vi "AlliGator Load I-m-phi Dataset.vi"(5 "Image Type":string="Image", 7 "Bkgd Image Subtraction?":bool, 8 "error in (no error)":errorcluster, 9 "Control References":T1, 10 "Folder Path":path, 11 "AlliGator IV DVR in":refnum<data-value>) -> (0 "error out":errorcluster, 2 "Folder Path (dup)":path, 3 "AlliGator IV DVR out":refnum<data-value>, 4 "Result String":string)   [LabVIEW 2021, in "AlliGator Files.lvlib"]
doc: "Loads a FLI dataset comprised of an intensity and phase image (FLIMBox)."
uses:
  AlliGator Files.lvlib
  AlliGator Internal Variables v2.ctl
  <vilib>/vision/Image Controls.llb/IMAQ Image.ctl
  AlliGator Gate Image Set.ctl
  AlliGator FLI Dataset Type.ctl
  AlliGator Data Series Type.ctl
  AlliGator Dataset Channel.ctl
  AlliGator Gate Arithmetic.ctl
  AlliGator Displayed Image.ctl
  Image/Named ROI Description.ctl
  AlliGator Decay Metadata v3.ctl
  AlliGator Decay Background Subtraction Info.ctl
  AlliGator Baseline Subtraction Method.ctl
  Graphs/XY Graph/XY Graph Plot Shift Parameters.ctl
  Graphs/XY Graph/XY Graph Plot Shift Method.ctl
  AlliGator Decay Extrapolation Parameters.ctl
  Phasor/Calibration Phasor (m, phi).ctl
  Phasor/Phasor Reference Series.ctl
  Phasor/Phasor Calibration Map v2.ctl
  Phasor/Phasor (g, s).ctl
  AlliGator Raw Phasor Plot Data v4.ctl
  Phasor/Phasor Standard Deviation Options.ctl
  AlliGator Phasor Multi-Harmonic Data.ctl
  Phasor/Phasor Harmonic Data.ctl
  AlliGator Decay Fit Options & Parameters v2.ctl
  Fits/IRF(X)PSED/Decay Fit Options v2.ctl
  Fits/Decay Convolution/Decay Model.ctl
  Fits/Residual Type.ctl
  Fits/IRF(X)PSED/Fit Weights Type.ctl
  Fits/Non-linear Fitting Method v2.ctl
  Fits/Fit Calculation Method.ctl
  Fits/Non-linear Fitting Algorithm.ctl
  AlliGator Decay Fit Parameter Constraints 2.ctl
  Fits/IRF(X)PSED/Decay Fit Parameters In List.ctl
  Fits/IRF(X)PSED/MLE Baseline Offset Type.ctl
  AlliGator Decay Preprocessing Parameters.ctl
  Fits/IRF(X)PSED/Decay Fit Parameters & Derived Quantities List.ctl
  AlliGator Dataset Ctrl Refnums.ctl
  AlliGator After Loading Dataset Information.ctl
  AlliGator Gate Images Structure.ctl
  AlliGator I-m-phi Component List.ctl
  089290e1-c93f-4b42-a3f3-b2d44885c075.vi
  Arrays/n x n Kernel Convolution (SGL).vi
  Arrays/n x n Smoothen Array (SGL) v3.vi
  Arrays/n x n Kernel Convolution (SGL).vi/d0ebc029-cbaa-4c82-a58c-923c59c440da.vi
  Arrays/n x n Kernel Convolution (SGL).vi/b80d5e79-a0c8-46e2-aba9-3d60e0093a16.vi
  <vilib>/Analysis/2dsp.llb/Convolution.vi
  <vilib>/Analysis/2dsp.llb/2D Convolution (DBL).vi
  Arrays/Truncate Kernel.vi
  Arrays/Replace NaN by 0 (2D SGL).vi
  Arrays/n x n Smoothen Array (SGL) v3.vi/d0ebc029-cbaa-4c82-a58c-923c59c440da.vi
  Arrays/n x n Smoothen Array (SGL) v3.vi/b80d5e79-a0c8-46e2-aba9-3d60e0093a16.vi
  Arrays/Replace NaN by 0 (2D SGL).vi/df975b44-f6c5-4554-af30-980613d33749.vi
  Time/High Resolution Timing.vi
  Arrays/Compute n x n Kernel (SGL).vi
  <vilib>/Utility/error.llb/Simple Error Handler.vi
  <vilib>/Utility/error.llb/Error Cluster From Error Code.vi
  <vilib>/ErrorRing/Error Ring.xnode
  Image/Image.lvlib
  AlliGator Source Image.lvlib
  AlliGator GUI.lvlib
  GUI/GUI.lvlib
  Boolean/Boolean.lvlib
  Error/Error.lvlib
  Arrays/Arrays.lvlib
  Strings/Strings.lvlib
  Phasor/Phasor.lvlib
  AlliGator Decay Preprocessing.lvlib
  Graphs/XY Graph/XY Graph Add-Ons.lvlib
  AlliGator Phasor Graph.lvlib
  AlliGator Internal Variables.lvlib
  AlliGator Phasor Plot.lvlib
  Fits/Fits.lvlib
  AlliGator Decay Fit.lvlib
  AlliGator Decay Fit Parameter Map.lvlib
  AlliGator Settings.lvlib
  AlliGator Dual-Channel Datasets.lvlib
panel:
  out "# disposed images":i32
  out "# created images":i32
  # "see the AlliGator License on the block diagram (Ctrl+E or Window:Show Block Diagram)"
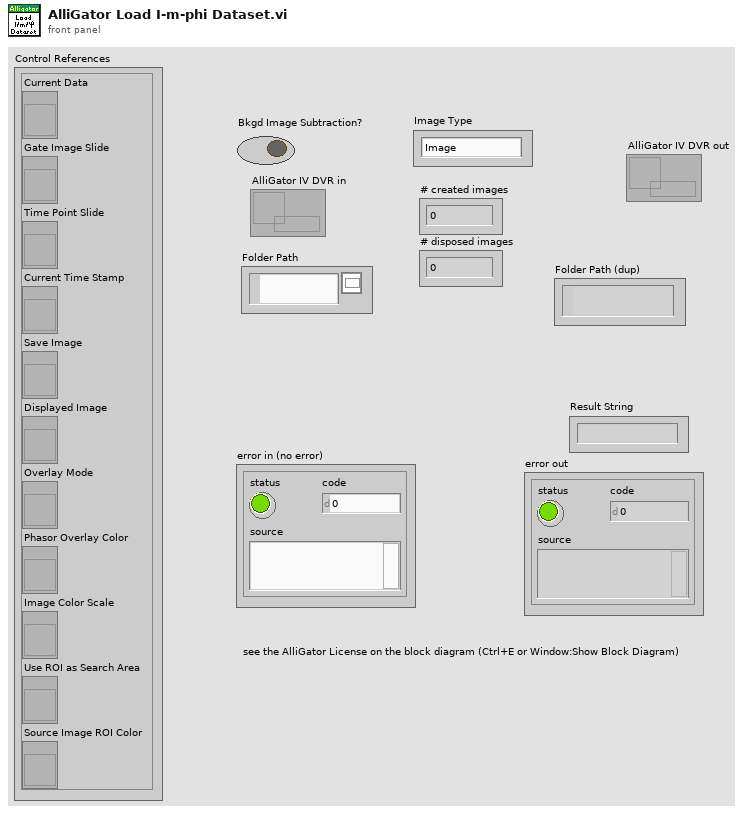
[diagram p1: front panel]
types:
  T1 = typedef "AlliGator GUI.lvlib/AlliGator Dataset Ctrl Refnums.ctl" = cluster{"Current Data":refnum<vi>, "Gate Image Slide":refnum<vi>, "Time Point Slide":refnum<vi>, "Current Time Stamp":refnum<vi>, "Save Image":refnum<vi>, "Displayed Image":refnum<vi>, "Overlay Mode":refnum<vi>, "Phasor Overlay Color":refnum<vi>, "Image Color Scale":refnum<vi>, "Use ROI as Search Area":refnum<vi>, "Source Image ROI Color":refnum<vi>}
  T2 = typedef "AlliGator Files.lvlib/AlliGator After Loading Dataset Information.ctl" = cluster{"Nanotime Gate Separation":dbl[unit], "Gate Width":dbl[unit], "Laser Period":dbl[unit], "Data Description":string, "# Pixel X":i32, "# Pixel Y":i32, "Gates to Use":cluster{"Start":u32, "End":u32}, "Gate Step":i32, "SYNC Period":dbl[unit], "X Binning":i32, "Y Binning":i32, "Gates to":bool, "Metadata":string, "Gate Image Exposure":dbl[unit], "Gate Image Integration":dbl[unit], "Macrotime Gate Separation":dbl[unit]}
  T3 = typedef "AlliGator Files.lvlib/AlliGator FLI Dataset Type.ctl" = enum16{"HDF5 FLI Dataset", "Gate Image Folder", ".sdt FLI Dataset (Becker & Hickl)", ".ptu FLI Dataset (PicoQuant)", "SS1 FLI Dataset", "SS2 FLI Dataset", "I/m/phi Dataset", ".bin FLI Dataset (PicoQuant Binned)", ".bin FLI Dataset (Piccolo Binned)"}
  T4 = typedef "AlliGator Files.lvlib/AlliGator Gate Images Structure.ctl" = cluster{"SGL Image Max":T5, "SGL Image Sum":T5, "SGL Gate Images":T5[], "SGL Image Min":T5}
  T5 = typedef "IMAQ Image.ctl" = refnum<image>
  T6 = typedef "AlliGator Files.lvlib/AlliGator I-m-phi Component List.ctl" = enum16{"Intensity", "g", "s"}
  T7 = typedef "FLIMBox.lvlib/FLIMbox Data.ctl" = cluster{"Software":string, "Base Frequency":dbl[unit], "X Size":i32, "Y Size":i32, "Metadata":string, "Intensity":sgl[][], "Harmonic Number":u8, "Harmonic Orders":u8[], "Harmonic Data":T8[], "File Version":string}
  T8 = typedef "FLIMBox.lvlib/FLIMbox Harmonic Data.ctl" = cluster{"Modulus":sgl[][], "Phase":sgl[][], "Harmonic Order":u8}
  T9 = typedef "AlliGator Source Image.lvlib/AlliGator Image Loading Options.ctl" = cluster{"Pixel Well Capacity":u32, "Pile-up Correction":bool, "Gate Step":i32, "Image Smoothing Options":T10, "Gates to Skip":T13, "File Background Subtraction":bool, "Background File Path":path, "Image Binning Options":T14, "# Gates":u32, "Gates to Keep":T15, "Define Gates to":bool, "Hot Pixel Removal":T16, "Dataset Scaling Factor":dbl}
  T10 = typedef "AlliGator Settings.lvlib/AlliGator Image Smoothing Options.ctl" = cluster{"Use Image Smoothing":bool, "Kernel Type":T11, "Bin":i32, "Algorithm":T12}
  T11 = typedef "Arrays.lvlib/Kernel Type.ctl" = enum16{"Uniform", "Bilinear", "Gaussian"}
  T12 = typedef "Arrays.lvlib/Smoothing Algorithm.ctl" = enum16{"Rapid", "Thorough"}
  T13 = typedef "AlliGator Decay Analysis.lvlib/AlliGator Gates to Skip.ctl" = cluster{"Start":u32, "End":u32}
  T14 = typedef "AlliGator Source Image.lvlib/AlliGator Image Binning Options.ctl" = cluster{"Use Image Binning":bool, "X Bin":i32, "Y Bin":i32}
  T15 = typedef "AlliGator Settings.lvlib/AlliGator Gates to Keep.ctl" = cluster{"First":u32, "Last":u32}
  T16 = typedef "SwissSPAD Live.lvlib/SwissSPAD Live_Image Display Options.ctl" = cluster{"Remove Screamers":bool, "Delta":sgl, "Equalize Histogram":bool, "Percentile":sgl, "Hot Pixel Mask Image":path, "Use Hot Pixel Mask":bool}
  T17 = typedef "AlliGator Internal Variables.lvlib/AlliGator Internal Variables v2.ctl" = cluster{"Displayed Image":T5, "White Light Image":T5, "Mask Image":T5, "ROI Mask Image":T5, "Current Dataset Images 1":T18, "Background Dataset Images 1":T18, "Current Dataset Images 2":T18, "Background Dataset Images 2":T18, "Current Dataset Arithmetic Images":T18, "Accumulated Dataset Images 1":T18, "Accumulated Dataset Images 2":T18, "Accumulated Dataset Arithmetic Images":T18, "Phasor Plot Image":T5, "Decay Fit Parameter Map Image":T5, "Single Data Point Path":path, "White Light Image Path":path, "Mask Image Path":path, "Time-Series Folder":path, "[Time-Series Paths]":path[], "Current Dataset":i32, "Single Dataset Type":T3, "Current Folder":string, "AlliGator Data Series Type":T19, "# Datasets":i32, "Dual-Channel Dataset":bool, "Selected Channel Name":string, "Dataset Channel":T20, "Channel Arithmetic":T21, "Dual-Channel Background Dataset":bool, "Background Channel":T20, "Dual-Channel Accumulated Dataset":bool, "Start Time":dbl, "[Time-Series Timestamps]":dbl[], "[Intensity Corrections]":dbl[], "Time Series Script":bool, "Type of Displayed Image":T22, "Gate Image Slide":u16, "# Gates":i32, "ROIs":T23[], "ROI Decay":cluster{"t Array":dbl[], "I Array":dbl[]}, "Valid Decay":bool, "Decay  Metadata":T25, "Reference Decay Plot Name":string, "Reference Decay":cluster{"t Array":dbl[], "I Array":dbl[]}, "Decay Shift Plot":cluster{"Time Stamps":dbl[], "Decay Shifts":dbl[]}, "[Decays Max Values]":sgl[], "[Decays Min Values]":sgl[], "Calibration Phasor":T31, "Calibration Phasor Series":T32, "Phasor Calibration Map":T33, "Calibration Map MD5 Digest":string, "Last Raw Phasor":T34, "Last Calibrated Phasor":T34, "Last Calibrated Phasor SDV":T34, "Phasor Graph:Phasor Plot":cluster{"g Array":dbl[], "s Array":dbl[]}, "Phasor Graph:Phasor SDV Plot":cluster{"g Array":dbl[], "s Array":dbl[]}, "[Phasor Graph:Raw Phasor Plots]":T35[], "Phasor Plot locked to Ref 1":i32, "[Phasor Plot(s) locked to Ref 1]":i32[], "[Phasor Plot(s) locked to Ref 2]":i32[], "[Pixel Phasors]":T34[], "[[Sum Image]]":dbl[][], "[[CSG Phasors]]":csg[][], "[[Valid Pixel?]]":bool[][], "I/m/phi Dataset":cluster{"I/m/phi Dataset?":bool, "Base Frequency":dbl[unit], "Harmonic Orders":u8[]}, "Multi Phasor Plot Data":T37, "Decay Fit Options & Parameters":T39, "Fit Options: Decay Preprocessing Parameters":T50, "Fit Options: Reference Decay":cluster{"t Array":dbl[], "I Array":dbl[]}, "Is Full Image Parameters Map":bool, "Is Single-Pixels Parameters Map":bool, "NLSF Parameters Map X Resolution":i32, "NLSF Parameters Map Y Resolution":i32, "[Single Decay Fit Parameters]":dbl[], "Fit Model":T41, "[[Multiple Decays Fit Parameters]]":dbl[][], "[[Multiple Decays Fit Parameter SDVs]]":dbl[][], "[[IRFs]]":dbl[][], "IRF Array Time Axis":dbl[], "Decay Array Time Axis":dbl[], "[Decay Fit Parameter Names]":T51[], "[[Phasor Ratios]]":dbl[][], "[[Average Lifetimes]]":dbl[][], "Amplitude Weighted Average Lifetime":bool, "[Decay Sum]":dbl[], "[[User-defined Quantities]]":dbl[][], "User-defined Quantity":string}
  T18 = typedef "AlliGator Files.lvlib/AlliGator Gate Image Set.ctl" = cluster{"SGL Image Max":T5, "SGL Image Sum":T5, "SGL Gate Images":T5[], "SGL Image Min":T5}
  T19 = typedef "AlliGator Files.lvlib/AlliGator Data Series Type.ctl" = enum16{"Not a Supported Series", "Gate Images Folder Series", "SwissSPAD 2 Dataset Series", "B&H FLI Dataset Series", "PicoQuant PTU FLI Dataset Series", "PicoQuant BIN FLI Dataset Series", "Piccolo hist BIN FLI Dataset Series", "HDF5 FLI Dataset Series"}
  T20 = typedef "AlliGator Dual-Channel Datasets.lvlib/AlliGator Dataset Channel.ctl" = enum16{"G2", "INT"}
  T21 = typedef "AlliGator Settings.lvlib/AlliGator Gate Arithmetic.ctl" = enum16{"None", "INT-G2", "G2/INT*<INT>", "(1 - G2/INT)*<INT>"}
  T22 = typedef "AlliGator Source Image.lvlib/AlliGator Displayed Image.ctl" = enum16{"Single Gate", "Sum of All Gates", "Max of All Gates", "Min of All Gates", "-", "White Ligth Image", "Mask Image"}
  T23 = typedef "Image.lvlib/Named ROI Description.ctl" = cluster{"ROI Descriptor":T24, "ROI Name":string, "Overlay Color":u32}
  T24 = typedef "ROI Descriptor" = cluster{"Global Rectangle":i32[], "Contours":cluster{"ID":enum32{"External", "Internal"}, "Type":u32, "Coordinates":i32[]}[]}
  T25 = typedef "AlliGator Phasor Graph.lvlib/AlliGator Decay Metadata v3.ctl" = cluster{"ROI Descriptor":T24, "ROI Center":cluster{"X":i32, "Y":i32}, "Decay Background Subtraction Info":T26, "Decay Reverted":bool, "Decay Smoothened":bool, "Decay Straightened":bool, "Fitted Tau (Decay Straightening)":dbl, "Decay Shift Parameters":T28, "Decay Shifted":bool, "Decay Extrapolated":bool, "Decay Extrapolation Parameters":T30, "Decay Normalized":bool, "Fold Decay":bool, "# Folds":u32}
  T26 = typedef "AlliGator Decay Analysis.lvlib/AlliGator Decay Preprocessing.lvlib/AlliGator Decay Background Subtraction Info.ctl" = cluster{"Laser Period":dbl[unit], "Gate Duration":dbl[unit], "Baseline Subtraction Method":T27, "Background Definition Range":cluster{"Min Gate":dbl[unit], "Max Gate":dbl[unit]}, "Total Intensity w/o Bkgd Subtraction":dbl, "Bkgd-subtracted Intensity (exp)":dbl, "# Data Points":i32, "Background/Gate":dbl, "Fitted Lifetime":dbl[unit], "Bkgd-subtracted Intensity (theo)":dbl}
  T27 = typedef "AlliGator Decay Analysis.lvlib/AlliGator Decay Preprocessing.lvlib/AlliGator Baseline Subtraction Method.ctl" = enum16{"Mean", "Min", "Square Gated Single-Exponential", "File", "Constant"}
  T28 = typedef "XY Graph Add-Ons.lvlib/XY Graph Plot Shift Parameters.ctl" = cluster{"Type":T29, "Shift":dbl[unit], "Threshold":dbl, "Rotate":bool}
  T29 = typedef "XY Graph Add-Ons.lvlib/XY Graph Plot Shift Method.ctl" = enum16{"Default", "CFD", "Threshold", "Cross-Correlation"}
  T30 = typedef "AlliGator Decay Analysis.lvlib/AlliGator Decay Preprocessing.lvlib/AlliGator Decay Extrapolation Parameters.ctl" = cluster{"Additional Points":u32, "Head Fraction":dbl, "Fitted Tau":dbl, "Use Periodicity":bool, "Use Cursors":bool, "Tail Fraction":dbl}
  T31 = typedef "Phasor.lvlib/Calibration Phasor (m, phi).ctl" = cluster{"m":dbl, "phi":dbl, "Phasor Frequency":dbl[unit], "Reference Lifetime":dbl[unit]}
  T32 = typedef "Phasor.lvlib/Phasor Reference Series.ctl" = cluster{"m Array":dbl[], "phi Array":dbl[], "Phasor Frequency":dbl[unit], "Calibration Lifetime":dbl[unit]}
  T33 = typedef "Phasor.lvlib/Phasor Calibration Map v2.ctl" = cluster{"Phasor Frequency":dbl[unit], "Calibration Lifetime":dbl[unit], "ROI Centers":cluster{"X":i32, "Y":i32}[], "ROI Descriptors":T24[], "Map Resolution X":i32, "Map Resolution Y":i32, "z Array":cdb[]}
  T34 = typedef "Phasor.lvlib/Phasor (g, s).ctl" = cluster{"g":dbl, "s":dbl}
  T35 = typedef "AlliGator Phasor Graph.lvlib/AlliGator Raw Phasor Plot Data v4.ctl" = cluster{"Phasor Plot Name":string, "Raw Phasor Plot":T34[], "Phasor Frequency":dbl[unit], "[Decay Metadata]":T25[], "Raw Phasor Plot SDV":T34[], "Phasor SDV Options":T36, "[Calibration Phasor]":T31[]}
  T36 = typedef "Phasor.lvlib/Phasor Standard Deviation Options.ctl" = cluster{"Compute Estimated SDV":bool, "# Replicas":u32, "Use Estimated Average Phasor":bool}
  T37 = typedef "AlliGator Phasor Plot.lvlib/AlliGator Phasor Multi-Harmonic Data.ctl" = cluster{"Base Frequency":dbl[unit], "# Harmonics":u8, "Harmonic Orders":u8[], "Phasor Plot Settings Checksum":u64, "Phasor Harmonic Data Array":T38[]}
  T38 = typedef "Phasor.lvlib/Phasor Harmonic Data.ctl" = cluster{"Phasor Harmonic Name":string, "Phasor Plot Settings Checksum":u64, "Phasor Frequency":dbl[unit], "Base Frequency":dbl[unit], "Harmonic Order":u8, "Phasor Plot Parameters":string, "Phasor Array [[CSG]]":csg[][], "Dataset File Path":path}
  T39 = typedef "AlliGator Decay Fit Parameter Map.lvlib/AlliGator Decay Fit Options & Parameters v2.ctl" = cluster{"SYNC Period":dbl[unit], "Fit Options":T40, "Fit Parameter Constraints":T47[], "MLE Baseline Offset":dbl, "MLE Baseline Offset Type":T49}
  T40 = typedef "Fits.lvlib/Decay Fit Options v2.ctl" = cluster{"Show Fit Residuals":bool, "Fit Model":T41, "Residual Type":T42, "Max Decay Percentile":dbl, "Min Decay Percentile":dbl, "Show Full Decay":bool, "Weights":T43, "Fitting Method":T44, "Compute Parameter Uncertainties":bool, "Periodic Boundaries":bool, "Model Calculation":T45, "Period":dbl[unit], "Termination Criteria":cluster{"Max Iterations":i32, "Max Function Calls":i32, "Max Time":dbl[unit], "Function Tolerance":dbl, "Parameter Tolerance":dbl, "Gradient Tolerance":dbl, "Min Lambda":dbl, "Max Lambda":dbl, "Initial Tick Count":u32}, "Offset Resolution":dbl[unit], "Use Local IRF":bool, "Fitting Algorithm":T46}
  T41 = typedef "Fits.lvlib/Decay Model.ctl" = enum16{"1-Exponential", "2-Exponentials"}
  T42 = typedef "Fits.lvlib/Residual Type.ctl" = enum16{"Standard", "Normalized", "Reduced"}
  T43 = typedef "Fits.lvlib/Fit Weights Type.ctl" = enum16{"Unweighted", "1/Variance", "Best of All"}
  T44 = typedef "Fits.lvlib/Non-linear Fitting Method v2.ctl" = enum16{"Least Square", "Least Absolute Residual", "Bisquare", "MLE", "-", "Best of All"}
  T45 = typedef "Fits.lvlib/Fit Calculation Method.ctl" = enum16{"Simulation", "Convolution", "Integration"}
  T46 = typedef "Fits.lvlib/Non-linear Fitting Algorithm.ctl" = enum16{"Levenberg-Marquardt", "Trust-Region Dogleg"}
  T47 = typedef "AlliGator Decay Analysis.lvlib/AlliGator Decay Fit.lvlib/AlliGator Decay Fit Parameter Constraints 2.ctl" = cluster{"Fit Parameter":T48, "Min Value":dbl, "Max Value":dbl, "Global":bool, "Used":bool}
  T48 = typedef "Fits.lvlib/Decay Fit Parameters In List.ctl" = enum16{"Offset", "Baseline", "A_1", "tau_1", "A_2", "tau_2"}
  T49 = typedef "Fits.lvlib/MLE Baseline Offset Type.ctl" = enum32{"Absolute", "Percentage"}
  T50 = typedef "AlliGator Decay Analysis.lvlib/AlliGator Decay Preprocessing.lvlib/AlliGator Decay Preprocessing Parameters.ctl" = cluster{"Background Subtraction":bool, "Straighten Decay":bool, "Reverse Gates":bool, "1-Normalized Decay":bool, "Smoothen Decay":bool, "Smoothing Parameter":dbl, "Shift Decay":bool, "Decay Shift Parameters":T28, "Extrapolate Decay":bool, "Additional Points":u32, "Head Fraction":dbl, "Pixel-Normalize Decay":bool, "Use Periodicity":bool, "Use Cursors":bool, "Tail Fraction":dbl, "Use Decay Pre-Processing":bool, "Fold Decay":bool, "# Folds":u32, "[0-1]-Normalized Decay":bool}
  T51 = typedef "Fits.lvlib/Decay Fit Parameters & Derived Quantities List.ctl" = enum16{"Offset", "Baseline", "A_1", "tau_1", "A_2", "tau_2", "<tau>_a", "f1_a", "f2_a", "<tau>_i", "f1_i", "f2_i", "-", "R^2", "Chi^2"}
  T52 = typedef "Image Type" = u32
  T53 = typedef "Image.lvlib/Image Characteristics.ctl" = cluster{"Calibration":T54, "File Type":string, "X Resolution":i32, "Y Resolution":i32, "File Data Type":i32, "Image Type":T52}
  T54 = typedef "Simple Grid Descriptor" = cluster{"X Step":sgl, "Y Step":sgl, "Unit":T55}
  T55 = typedef "Image Unit" = enum32{"Undefined", "Angström", "Micrometer", "Millimeter", "Centimeter", "Meter", "Kilometer", "Microinch", "Inch", "Feet", "Nautical miles", "Standard miles", "Steps"}
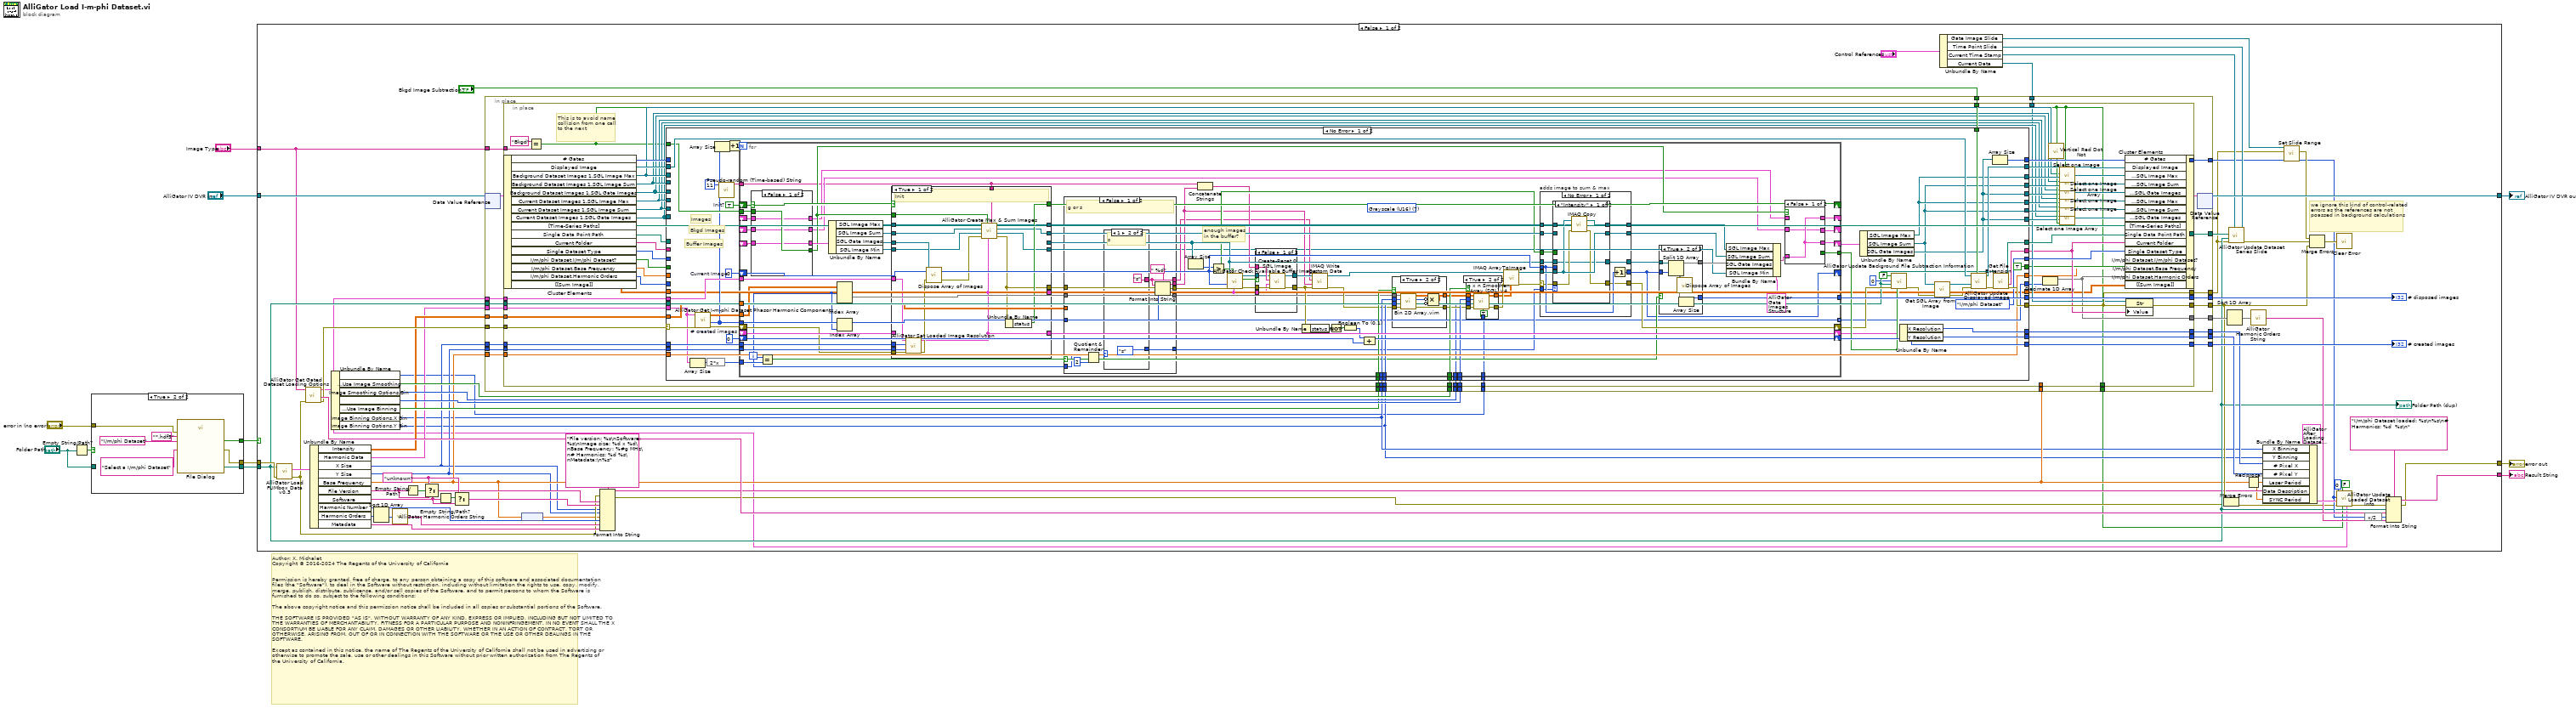
[diagram p0: block diagram]
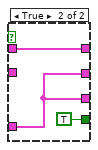
[diagram p2: hidden frame]
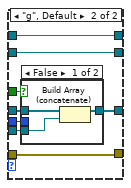
[diagram p6: hidden frame]
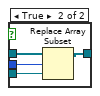
[diagram p7: hidden frame]
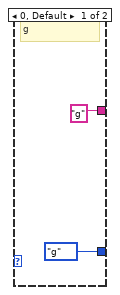
[diagram p10: hidden frame]
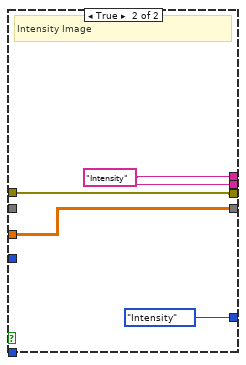
[diagram p11: hidden frame]
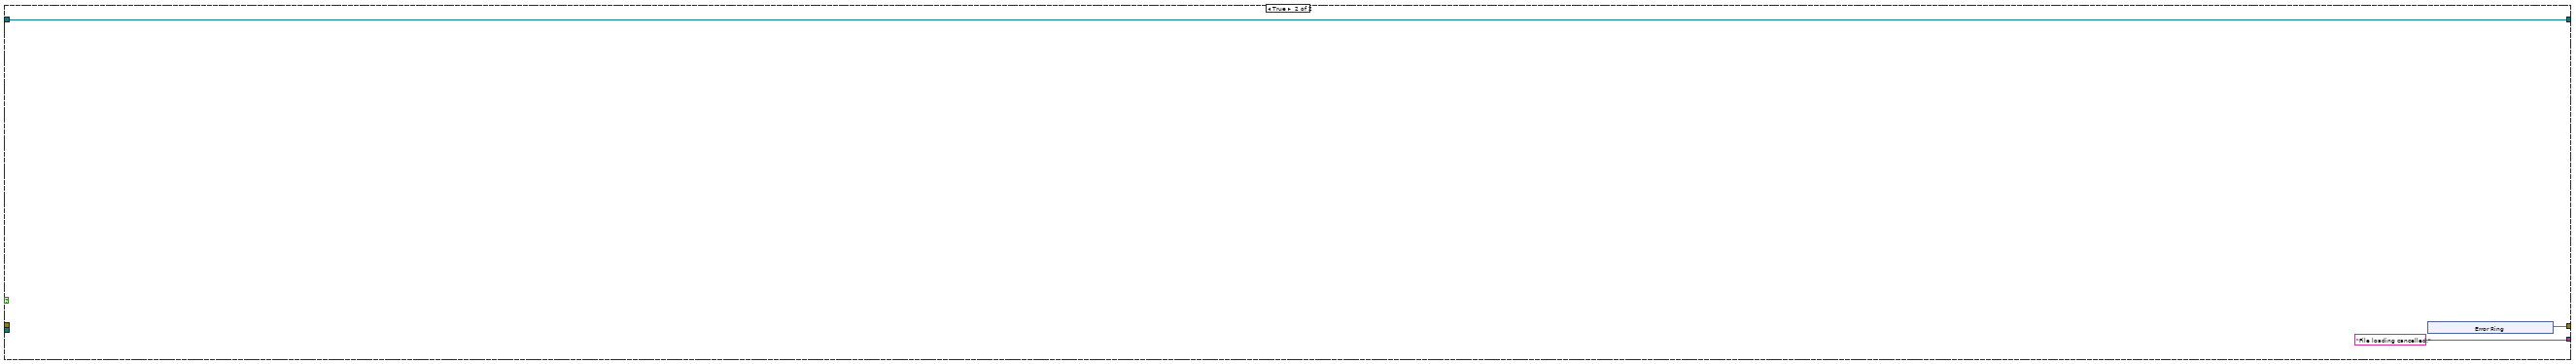
[diagram p16: hidden frame]
diagram:
  # "Author: X. Michalet\nCopyright © 2016-2024 The Regents of the University of California\n \n\nPermission is hereby granted, free of charge, to any person obtaining a copy of this software and associated documentation files (the \"Software\"), to deal in the Software without restriction, including without limitation the rights to use, copy, modify, merge, publish, distribute, sublicense, and/or sell copies of the Software, and to permit persons to whom the Software is furnished to do so, subject to the following conditions:\n\nThe above copyright notice and this permission notice shall be included in all copies or substantial portions of the Software.\n\nTHE SOFTWARE IS PROVIDED \"AS IS\", WITHOUT WARRANTY OF ANY KIND, EXPRESS OR IMPLIED, INCLUDING BUT NOT LIMITED TO THE WARRANTIES OF MERCHANTABILITY, FITNESS FOR A PARTICULAR PURPOSE AND NONINFRINGEMENT. IN NO EVENT SHALL THE X CONSORTIUM BE LIABLE FOR ANY CLAIM, DAMAGES OR OTHER LIABILITY, WHETHER IN AN ACTION OF CONTRACT, TORT OR OTHERWISE, ARISING FROM, OUT OF OR IN CONNECTION WITH THE SOFTWARE OR THE USE OR OTHER DEALINGS IN THE SOFTWARE.\n\nExcept as contained in this notice, the name of The Regents of the University of California shall not be used in advertising or otherwise to promote the sale, use or other dealings in this Software without prior written authorization from The Regents of the University of California."
  n1 = Empty String/Path?(string/path="Folder Path") -> (empty?=w7:bool)
  n2 = case shown="True" w7 {
    tunnel: "error in (no error)" -> [w12 w20]
    tunnel: [w13 w17] -> w4
    tunnel: [w12 w16] -> w3
    tunnel: "Folder Path" -> [w13 _]
    tunnel: [_ w15] -> w2
    frame False {
    }
    frame True {
      n3 = call "File Dialog"("prompt"="Select a I/m/phi Dataset", "error in"=w20, "pattern (all files)"="*.hdf5", "pattern label"="I/m/phi Dataset") -> ("selected path"=w17:path, "cancelled"=w15:bool, "error out"=w16:errorcluster)  [unwired: 8 in, 1 out]
    }
  }
  n4 = case shown="False" w2 {
    tunnel: [w88 "File loading cancelled."] -> w11
    tunnel: [w70 w478] -> w10
    tunnel: "AlliGator IV DVR in" -> [w77 w477]
    tunnel: [w76 w477] -> w8
    tunnel: w4 -> [w52 _]
    tunnel: w3 -> [w63 _]
    tunnel: "Image Type" -> [w24 _]
    frame False {
      w43 = "unknown" ("t")
      # "we ignore this kind of control-related errors as the references are not poassed in background calculations"
      n5 = call "AlliGator Load FLIMbox Data v0.3.vi"("Error In"=w63, "File Path"=w52) -> ("Error Out"=w37:errorcluster, "FLIMbox Data out"=w53:T7)  [unwired: 8 in]
      n6 = call "AlliGator Get Gated Dataset Loading Options.vi"("error in (no error)"=w37, "Image Type"=w24) -> ("error out"=w64:errorcluster, "Dataset Loading Options string"=w82:string, "Dataset Loading Options"=w21:T9)  [unwired: 6 in, 1 out]
      n7 = Unbundle By Name(w53) -> ("Intensity"=w62:sgl[][], "Harmonic Data"=w61:T8[], "X Size"=w29:i32, "Y Size"=w28:i32, "Base Frequency"=w31:dbl[unit], "File Version"=w46:string, "Software"=w44:string, "Harmonic Number"=w40:u8, "Harmonic Orders"=w49:u8[], "Metadata"=w38:string)
      n8 = Unbundle By Name(w21) -> ("Image Smoothing Options.Algorithm"=w23:T12, "Image Smoothing Options.Use Image Smoothing"=w79:bool, "Image Smoothing Options.Bin"=w81:i32, "Image Smoothing Options.Kernel Type"=w80:T11, "Image Binning Options.Use Image Binning"=w78:bool, "Image Binning Options.X Bin"=w26:i32, "Image Binning Options.Y Bin"=w25:i32)
      n9 = Sort 1D Array(array=w49) -> (sorted array=w50:u8[])
      n10 = call "AlliGator Harmonic Orders String.vi"("Harmonic Order Array"=w50) -> ("String"=w39:string)  [unwired: 8 in]
      n11 = Empty String/Path?(string/path=w46) -> (empty?=w47:bool)
      n12 = Select(t=w43, s=w47, f=w46) -> (s? t:f=w42:string)
      n13 = Empty String/Path?(string/path=w44) -> (empty?=w45:bool)
      n14 = Select(t=w43, s=w45, f=w44) -> (s? t:f=w41:string)
      n15 = node(w31) -> (w30:dbl)
      n16 = Format Into String(format string="File version: %s\nSoftware: %s\nImage size: %d x %d\nBase Frequency: %#g MHz\n# Harmonics: %d %s\nMetadata:\n%s", error in=w37, w42, w41, w29, w28, w30, w40, w39, w38) -> (resulting string=w32:string, error out=w36:errorcluster)  [unwired: 1 in]
      n17 = Unbundle By Name("Control References") -> ("Gate Image Slide"=w72:refnum<vi>, "Time Point Slide"=w73:refnum<vi>, "Current Time Stamp"=w74:refnum<vi>, "Current Data"=w67:refnum<vi>)
      n18 = in-place {
        in-place-border: [w121] -> w90
        in-place-border: w24 -> [w120]
        in-place-border: [w119] -> w87
        in-place-border: [w118] -> w60
        in-place-border: [w117] -> w59
        in-place-border: w64 -> [w116]
        in-place-border: "Bkgd Image Subtraction?" -> [w115]
        in-place-border: [w114] -> w65
        in-place-border: w81 -> [w113]
        in-place-border: w80 -> [w112]
        in-place-border: w79 -> [w111]
        in-place-border: [w110] -> w35
        in-place-border: w78 -> [w109]
        in-place-border: w26 -> [w108]
        in-place-border: w25 -> [w107]
        in-place-border: w21 -> [w106]
        in-place-border: [w96] -> w71
        in-place-border: w67 -> [w103]
        in-place-border: [w102] -> w34
        in-place-border: w62 -> [w101]
        in-place-border: w61 -> [w100]
        in-place-border: w29 -> [w99]
        in-place-border: w28 -> [w98]
        in-place-border: w52 -> [w97]
        in-place-border: w31 -> [w95]
        in-place-border: w31 -> [w94]
        in-place-border: [w93] -> w54
        in-place-border: w23 -> [w92]
        in-place-border: [w91] -> w22
        n19 = in-place-dvr #1(w77) -> (w105:T17)  [unwired: 1 out]
        n20 = in-place {
          in-place-border: [w186] -> w121
          in-place-border: w120 -> [w163]
          in-place-border: [w185] -> w119
          in-place-border: [w184] -> w118
          in-place-border: [w183] -> w117
          in-place-border: w116 -> [w182]
          in-place-border: w115 -> [w181]
          in-place-border: [w173] -> w114
          in-place-border: w113 -> [w180]
          in-place-border: w112 -> [w179]
          in-place-border: w111 -> [w178]
          in-place-border: [w143] -> w110
          in-place-border: w109 -> [w177]
          in-place-border: w108 -> [w176]
          in-place-border: w107 -> [w175]
          in-place-border: w106 -> [w174]
          in-place-border: w103 -> [w142]
          in-place-border: [w140] -> w102
          in-place-border: w101 -> [w139]
          in-place-border: w100 -> [w138]
          in-place-border: w99 -> [w137]
          in-place-border: w98 -> [w136]
          in-place-border: w97 -> [w135]
          in-place-border: [w134] -> w96
          in-place-border: w95 -> [_]
          in-place-border: w94 -> [w128]
          in-place-border: [w126] -> w93
          in-place-border: w92 -> [w125]
          in-place-border: [w122] -> w91
          # "This is to avoid name collision from one call to the next"
          n21 = in-place-cluster #2(w105) -> ("# Gates"=w171:i32, "Displayed Image"=w170:T5, "Background Dataset Images 1.SGL Image Max"=w149:T5, "Background Dataset Images 1.SGL Image Sum"=w148:T5, "Background Dataset Images 1.SGL Gate Images"=w147:T5[], "Current Dataset Images 1.SGL Image Max"=w146:T5, "Current Dataset Images 1.SGL Image Sum"=w145:T5, "Current Dataset Images 1.SGL Gate Images"=w144:T5[], "[Time-Series Paths]"=w134:path[], "Single Data Point Path"=w168:path, "Current Folder"=w167:string, "Single Dataset Type"=w166:T3, "I/m/phi Dataset.I/m/phi Dataset?"=w132:bool, "I/m/phi Dataset.Base Frequency"=w131:dbl[unit], "I/m/phi Dataset.Harmonic Orders"=w130:u8[], "[[Sum Image]]"=w124:dbl[][])
          n22 = Equal?(x="Bkgd", y=w163) -> (x = y?=w122:bool)
          n23 = case shown="No Error" w182 {
            selector: w182 -> [w203 w474]
            tunnel: [w240 _] -> w186
            tunnel: w122 -> [w217 _]
            tunnel: [w239 _] -> w185
            tunnel: [w238 _] -> w184
            tunnel: [w237 _] -> w183
            tunnel: w181 -> [w235 _]
            tunnel: [w231 w476] -> w173
            tunnel: w180 -> [w230 _]
            tunnel: w179 -> [w229 _]
            tunnel: w178 -> [w228 _]
            tunnel: [w220 w474] -> w143
            tunnel: w177 -> [w227 _]
            tunnel: w176 -> [w226 _]
            tunnel: w175 -> [w225 _]
            tunnel: w174 -> [w224 _]
            tunnel: [w223 w475] -> w172
            tunnel: w171 -> [_ w476]
            tunnel: w170 -> [w222 w475]
            tunnel: [w219 w472] -> w169
            tunnel: [w214 w473] -> w141
            tunnel: w168 -> [_ w472]
            tunnel: w167 -> [_ w473]
            tunnel: w166 -> [_ w471]
            tunnel: [AlliGator_FLI_Dataset_Type."I/m/phi Dataset" ("Single Dataset Type") w471] -> w165
            tunnel: [w215 w470] -> w159
            tunnel: [w191 w469] -> w156
            tunnel: [w216 w468] -> w153
            tunnel: [w216 w465] -> w152
            tunnel: [w191 w466] -> w151
            tunnel: [w215 w467] -> w150
            tunnel: w149 -> [_ w470]
            tunnel: w148 -> [_ w469]
            tunnel: w147 -> [_ w468]
            tunnel: w146 -> [_ w467]
            tunnel: w145 -> [_ w466]
            tunnel: w144 -> [_ w465]
            tunnel: w139 -> [w205 _]
            tunnel: w138 -> [w198 _]
            tunnel: w137 -> [w211 _]
            tunnel: w136 -> [w210 _]
            tunnel: w135 -> [w209 _]
            tunnel: [w208 w462] -> w127
            tunnel: [TRUE ("I/m/phi Dataset.I/m/phi Dataset?") w464] -> w133
            tunnel: w132 -> [_ w464]
            tunnel: w131 -> [_ w463]
            tunnel: w130 -> [_ w462]
            tunnel: [w206 w463] -> w129
            tunnel: w128 -> [w206 _]
            tunnel: w125 -> [w197 _]
            tunnel: w124 -> [w195 w461]
            tunnel: [w194 w461] -> w123
            frame No Error {
              w241 = 0  # # created images
              w242 = 0  # Current Image
              w243 = TRUE  # Init?
              # "Images"
              # "Bkgd Images"
              # "Buffer Images"
              n24 = Array Size(array=w198) -> (size(s)=w213:i32)
              n25 = call "AlliGator Get I-m-phi Dataset Phasor Harmonic Components.vi"("Error In"=w203, "Harmonic Data"=w198) -> ("Error Out"=w202:errorcluster, "Harmonic Order"=w201:u8[], "Phasor Components"=w204:sgl[][][])  [unwired: 7 in]
              n26 = expression code="2*x"(w213) -> (w212:i32)
              n27 = Array Size(array=w201) -> (size(s)=w200:i32)
              n28 = call "Pseudo-random (Time-based) String.vi"("Length (10)"=u32 11) -> ("result string"=w196:string)  [unwired: 9 in, 1 out]
              n29 = Increment(x=w200) -> (x+1=w199:i32)
              n30 = for {
                N: w199 -> [_]
                shift-right: [w257] -> w232
                shift-left: w202 -> [w286]
                shift-right: [w311] -> _
                shift-left: _ -> [w321]
                shift-right: [w310] -> _
                shift-left: w243 -> [w322]
                shift-right: [w245] -> _
                shift-left: w242 -> [w325]
                shift-right: [w324] -> w240
                shift-left: w241 -> [w263]
                tunnel: w217 -> [w317]
                shift-right: [w313] -> w236
                shift-left: _ -> [w319]
                shift-right: [w312] -> _
                shift-left: _ -> [w320]
                tunnel: w196 -> [w247]
                tunnel: w212 -> [w323]
                tunnel: [w314] -> w239
                tunnel: [w307] -> w234
                shift-right: [w306] -> w233
                shift-left: _ -> [w305]
                tunnel: w230 -> [w249]
                tunnel: w229 -> [w302]
                tunnel: w228 -> [w301]
                tunnel: w227 -> [w300]
                tunnel: w226 -> [w299]
                tunnel: w225 -> [w298]
                tunnel: w224 -> [w297]
                tunnel: w205 -> [w268]
                tunnel: w211 -> [w288]
                tunnel: w210 -> [w287]
                tunnel: [w251] -> w208 mode=indexing
                tunnel: w204 -> [w254]
                tunnel: w201 -> [w256]
                tunnel: w197 -> [w248]
                i -> [w250]
                (unwired) T52 7 items=["Grayscale (U8)", "Grayscale (I16)", "Grayscale (SGL)", "Complex (CSG)", "RGB (U32)", "HSL (U32)", "RGB (U64)", "Grayscale (U16)"] ("Image Type")
                # "enough images in the buffer?"
                n31 = case shown="False" w322 {
                  tunnel: w317 -> [w450 w456]
                  tunnel: [w450 w456] -> w304
                  tunnel: w321 -> [w449 w453]
                  tunnel: w320 -> [w448 w454]
                  tunnel: w319 -> [w447 _]
                  tunnel: [w449 w452] -> w270
                  tunnel: [w448 w451] -> w271
                  tunnel: [w447 w455] -> w318
                  frame False {
                  }
                  frame True {
                    n32 = case shown="False" w456 {
                      tunnel: [w458 w459] -> w455
                      tunnel: w454 -> [w457 w459]
                      tunnel: w453 -> [w458 w460]
                      tunnel: [w458 w460] -> w452
                      tunnel: [w457 w459] -> w451
                      frame False {
                      }
                      frame True {
                      }
                    }
                  }
                }
                n33 = Equal?(x=w250, y=w323) -> (x = y?=w255:bool)
                n34 = Unbundle By Name(w318) -> ("SGL Image Max"=w295:T5, "SGL Image Sum"=w294:T5, "SGL Gate Images"=w291:T5[], "SGL Image Min"=w246:T5)
                n35 = Index Array(array=w254, index (dim 0)=w250) -> (element=w252:sgl[][])  [unwired: 2 in]
                n36 = Index Array(array=w256, index=w250) -> (element=w251:u8)
                n37 = case shown="True" w322 {
                  selector: w322 -> [_ w446]
                  tunnel: [w426 w444] -> w293
                  tunnel: w286 -> [w437 w442]
                  tunnel: [w439 w446] -> w310
                  tunnel: [w427 w445] -> w292
                  tunnel: w304 -> [w429 _]
                  tunnel: w295 -> [w432 w445]
                  tunnel: w294 -> [w431 w444]
                  tunnel: [w428 w441] -> w289
                  tunnel: w305 -> [_ w441]
                  tunnel: [w424 w442] -> w267
                  tunnel: w291 -> [w438 w443]
                  tunnel: [_ w443] -> w290
                  tunnel: w297 -> [w436 _]
                  tunnel: [w428 w441] -> w306
                  tunnel: w288 -> [w435 _]
                  tunnel: w287 -> [w434 _]
                  tunnel: w247 -> [w430 _]
                  tunnel: w246 -> [w423 w440]
                  tunnel: [w422 w440] -> w244
                  frame True {
                    # "Init"
                    n38 = call "AlliGator Set Loaded Image Resolution.vi"("Error In"=w437, "Image Y"=w434, "Image X"=w435, "Image Loading Options"=w436) -> ("Error Out"=w433:errorcluster, "Image Characteristics"=w428:T53)  [unwired: 6 in]
                    n39 = call "Dispose Array of Images.vi"("Array of Images"=w438, "error in (no error)"=w433) -> ("error out"=w425:errorcluster)  [unwired: 7 in]
                    n40 = call "AlliGator Create Max & Sum Images.vi"("Prefix"=w430, "Image Characteristics"=w428, "Image Type"=w429, "Error In"=w425, "Image Min"=w423, "Image Max"=w431, "Image Sum"=w432) -> ("Error Out"=w424:errorcluster, "Image Min"=w422:T5, "Image Max"=w426:T5, "Image Sum"=w427:T5)  [unwired: 1 in]
                    n41 = Unbundle By Name(w424) -> ("status"=w439:bool)
                  }
                  frame False {
                  }
                }
                n42 = case shown="False" w255 {
                  tunnel: [w411 w421] -> w260
                  tunnel: w251 -> [w409 _]
                  tunnel: [w408 w421] -> w261
                  tunnel: w267 -> [w407 w420]
                  tunnel: [w406 w420] -> w266
                  tunnel: w268 -> [_ w419]
                  tunnel: [w405 AlliGator_I-m-phi_Component_List."Intensity"] -> w259
                  tunnel: w250 -> [w404 _]
                  tunnel: w252 -> [w403 _]
                  tunnel: [w403 w419] -> w253
                  frame False {
                    # "g or s"
                    n43 = Quotient & Remainder(x=w404, y=2) -> (x-y*floor(x/y)=w412:i32)  [unwired: 1 out]
                    n44 = case shown="1" w412 {
                      tunnel: ["g" ("Key") "s" ("Key")] -> w411
                      tunnel: [AlliGator_I-m-phi_Component_List."g" AlliGator_I-m-phi_Component_List."s"] -> w405
                      frame 0, Default {
                        # "g"
                      }
                      frame 1 {
                        # "s"
                      }
                    }
                    n45 = Format Into String(format string=" %d", initial string=w411, error in=w407, w409) -> (resulting string=w408:string, error out=w406:errorcluster)
                  }
                  frame True {
                    w421 = "Intensity" ("Key")
                    # "Intensity Image"
                  }
                }
                n46 = Array Size(array=w290) -> (size(s)=w285:i32)
                n47 = Concatenate Strings(w247, w261) -> (w278:string)
                n48 = Greater?(x=w285, y=w325) -> (0:w284:bool)
                n49 = call "AlliGator Check Available Buffer Image.vi"("Image Characteristics"=w289, "Buffer Image available?"=w284, "error in (no error)"=w266, "Current Gate"=w325, "Image Buffer"=w290) -> ("error out"=w274:errorcluster, "Image Reused?"=w276:bool, "Gate Image"=w277:T5)  [unwired: 3 in, 1 out]
                n50 = case shown="False" w276 {
                  tunnel: w278 -> [w400 _]
                  tunnel: w277 -> [w399 w402]
                  tunnel: [w398 w402] -> w275
                  tunnel: w274 -> [w397 w401]
                  tunnel: [w396 w401] -> w265
                  tunnel: w289 -> [w395 _]
                  frame False {
                    n51 = call "Create-Reset 0 SGL Image.vi"("Error In"=w397, "Image Characteristics"=w395, "Image Name"=w400, "Image"=w399) -> ("Error Out"=w396:errorcluster, "New Image"=w398:T5)  [unwired: 6 in]
                  }
                  frame True {
                  }
                }
                n52 = Unbundle By Name(w265) -> ("status"=w273:bool)
                n53 = call "IMAQ Write Custom Data"("error in (no error)"=w265, "Custom Data In"=w261, "Key"=w260, "Image"=w275) -> ("error out"=w264:errorcluster, "Image Out"=w269:T5)  [unwired: 6 in]
                n54 = Not(x=w273) -> (.not. x?=w272:bool)
                n55 = Boolean To (0,1)(Boolean=w272) -> (0, 1=w262:i16)
                n56 = Compound Arithmetic op=ADD(w262, w263) -> (w324:i32)
                n57 = case shown="True" w300 {
                  tunnel: w264 -> [w347 w355]
                  tunnel: [w347 w354] -> w283
                  tunnel: w299 -> [_ w350]
                  tunnel: w298 -> [_ w349]
                  tunnel: w253 -> [w348 w353]
                  tunnel: [w348 w351] -> w282
                  frame False {
                  }
                  frame True {
                    n58 = call "Bin 2D Array.vim"("Error In"=w355, "Y Bin (1)"=w349, "X Bin (1)"=w350, "Array"=w353) -> ("Error Out"=w354:errorcluster, "Binned Array"=w352:sgl[][])  [unwired: 2 in, 4 out]
                    n59 = Compound Arithmetic op=MULTIPLY(w352, invert w350, invert w349) -> (w351:dbl[][])
                  }
                }
                n60 = case shown="True" w301 {
                  tunnel: w283 -> [w337 w346]
                  tunnel: [w337 w345] -> w281
                  tunnel: [w338 w344] -> w280
                  tunnel: w282 -> [w338 w343]
                  tunnel: w302 -> [_ w341]
                  tunnel: w249 -> [_ w340]
                  tunnel: w248 -> [_ w339]
                  frame False {
                  }
                  frame True {
                    n61 = call "n x n Smoothen Array (SGL) v4.vi"("Average"=TRUE, "Algorithm"=w339, "Error In"=w346, "Kernel Size"=w340, "Kernel Type"=w341, "Array in"=w343) -> ("Error Out"=w345:errorcluster, "Array out"=w344:sgl[][])  [unwired: 3 in, 1 out]
                  }
                }
                n62 = call "IMAQ ArrayToImage"("Image Pixels (Float)"=w280, "error in (no error)"=w281, "Image"=w269) -> ("error out"=w258:errorcluster, "Image Out"=w279:T5)  [unwired: 7 in]
                n63 = case "adds image to sum & max" shown="No Error" w258 {
                  selector: w258 -> [w357 w390]
                  tunnel: w293 -> [w361 w394]
                  tunnel: [w360 w394] -> w308
                  tunnel: w279 -> [w366 _]
                  tunnel: w284 -> [w368 _]
                  tunnel: w290 -> [w367 w393]
                  tunnel: w325 -> [w364 w392]
                  tunnel: [w365 w393] -> w316
                  tunnel: [w363 w392] -> w245
                  tunnel: w292 -> [w358 w391]
                  tunnel: [w359 w391] -> w309
                  tunnel: w259 -> [w362 _]
                  tunnel: [w356 w390] -> w257
                  frame No Error {
                    n64 = case shown="\"Intensity\"" w362 {
                      tunnel: w368 -> [_ w382]
                      tunnel: w367 -> [w369 w381]
                      tunnel: w366 -> [w374 w380]
                      tunnel: [w369 w379] -> w365
                      tunnel: w364 -> [_ w378]
                      tunnel: w361 -> [_ w376]
                      tunnel: [w374 w376] -> w360
                      tunnel: [w370 w377] -> w359
                      tunnel: w358 -> [w373 w377]
                      tunnel: w357 -> [w372 w375]
                      tunnel: [w371 w375] -> w356
                      frame "Intensity" {
                        n65 = call "IMAQ Copy"("error in (no error)"=w372, "Image Dst"=w373, "Image Src"=w374) -> ("error out"=w371:errorcluster, "Image Dst Out"=w370:T5)  [unwired: 3 in]
                      }
                      frame "g", Default {
                        n66 = case shown="False" w382 {
                          tunnel: w381 -> [w385 w389]
                          tunnel: w380 -> [w384 w388]
                          tunnel: w378 -> [_ w386]
                          tunnel: [w383 w387] -> w379
                          frame False {
                            n67 = Build Array (concatenate)(w385, w384) -> (w383:T5[])
                          }
                          frame True {
                            n68 = Replace Array Subset(array=w389, new element=w388, index=w386) -> (w387:T5[])
                          }
                        }
                      }
                    }
                    n69 = Increment(x=w364) -> (x+1=w363:i32)
                  }
                  frame Error {
                  }
                }
                n70 = case shown="True" w255 {
                  tunnel: w316 -> [w331 w336]
                  tunnel: [w331 w334] -> w315
                  tunnel: w245 -> [_ w335]
                  tunnel: [_ w332] -> w314
                  frame False {
                  }
                  frame True {
                    n71 = Split 1D Array(array=w336, index=w335) -> (first subarray=w334:T5[], second subarray=w333:T5[])
                    n72 = call "Dispose Array of Images.vi"("Array of Images"=w333) -> ()  [unwired: 8 in, 1 out]
                    n73 = Array Size(array=w333) -> (size(s)=w332:i32)
                  }
                }
                n74 = Bundle By Name(cluster=T4 {"SGL Image Max"=refnum, "SGL Image Sum"=refnum, "SGL Gate Images"=[], "SGL Image Min"=refnum} ("Images"), "SGL Image Max"=w309, "SGL Image Sum"=w308, "SGL Gate Images"=w315, "SGL Image Min"=w244) -> (w303:T4)
                n75 = case shown="False" w304 {
                  tunnel: [_ TRUE ("Init?")] -> w307
                  tunnel: [w326 w328] -> w312
                  tunnel: w303 -> [w327 w328]
                  tunnel: [w327 w329] -> w311
                  tunnel: w270 -> [_ w329]
                  tunnel: [w327 w328] -> w313
                  tunnel: w271 -> [w326 _]
                  frame False {
                  }
                  frame True {
                  }
                }
              }
              n76 = Unbundle By Name(w236) -> ("SGL Image Max"=w215:T5, "SGL Image Sum"=w191:T5, "SGL Gate Images"=w216:T5[])
              n77 = call "AlliGator Update Background File Subtraction Information.vi"("Background subtracted"=w234, "Error In"=w232, "Background Dataset Path"=w209, "Background Pixel Well Capacity"=u32 0, "Background Pile-up Correction"=FALSE) -> ("Error Out"=w193:errorcluster)  [unwired: 6 in]
              n78 = Unbundle By Name(w233) -> ("X Resolution"=w238:i32, "Y Resolution"=w237:i32)
              n79 = call "Get SGL Array from Image.vi"("error in (no error)"=w193, "Image Array in (Empty)"=w195, "Image Refnum in"=w191) -> ("error out"=w192:errorcluster, "Image Array out"=w194:dbl[][], "Image Refnum dup"=w190:T5)  [unwired: 6 in]
              n80 = call "AlliGator Update Displayed Image.vi"("Bkgd Image Subtraction?"=w235, "Error In"=w192, "Sum Image Ref"=w190, "Displayed Image Ref"=w222) -> ("Error Out"=w221:errorcluster, "Displayed Image Ref"=w223:T5)  [unwired: 6 in]
              n81 = Array Size(array=w216) -> (size(s)=w231:i32)
              n82 = call <vilib>:"Get File Extension.vi"("error in (no error)"=w221, "file"=w209) -> ("error out"=w220:errorcluster, "filename without extension"=w214:string, "dup file"=w219:path)  [unwired: 5 in, 2 out]
            }
            frame Error {
            }
          }
          n83 = Decimate 1D Array(w127) -> (w126:u8[])  [unwired: 1 out]
          n84 = call "Vertical Red Dot Not.vi"("B"=w122) -> ("Not(B)"=w154:bool)  [unwired: 8 in]
          n85 = call "Select one Image.vi"("Previous Image (F)"=w149, "New Image (T)"=w159, "Image to use"=w122) -> ("Selected Image"=w162:T5)  [unwired: 4 in]
          n86 = call "Select one Image.vi"("Previous Image (F)"=w148, "New Image (T)"=w156, "Image to use"=w122) -> ("Selected Image"=w161:T5)  [unwired: 4 in]
          n87 = call "Select one Image Array.vi"("Previous Images (F)"=w147, "New Images (T)"=w153, "Image to use"=w122) -> ("Selected Images"=w160:T5[])  [unwired: 4 in]
          n88 = call "Select one Image.vi"("Previous Image (F)"=w146, "New Image (T)"=w150, "Image to use"=w154) -> ("Selected Image"=w158:T5)  [unwired: 4 in]
          n89 = call "Select one Image.vi"("Previous Image (F)"=w145, "New Image (T)"=w151, "Image to use"=w154) -> ("Selected Image"=w157:T5)  [unwired: 4 in]
          n90 = call "Select one Image Array.vi"("Previous Images (F)"=w144, "New Images (T)"=w152, "Image to use"=w154) -> ("Selected Images"=w155:T5[])  [unwired: 4 in]
          n91 = in-place-cluster #2("# Gates"=w173, "Displayed Image"=w172, "Background Dataset Images 1.SGL Image Max"=w162, "Background Dataset Images 1.SGL Image Sum"=w161, "Background Dataset Images 1.SGL Gate Images"=w160, "Current Dataset Images 1.SGL Image Max"=w158, "Current Dataset Images 1.SGL Image Sum"=w157, "Current Dataset Images 1.SGL Gate Images"=w155, "[Time-Series Paths]"=w134, "Single Data Point Path"=w169, "Current Folder"=w141, "Single Dataset Type"=w165, "I/m/phi Dataset.I/m/phi Dataset?"=w133, "I/m/phi Dataset.Base Frequency"=w129, "I/m/phi Dataset.Harmonic Orders"=w126, "[[Sum Image]]"=w123) -> (w104:T17)
          n92 = property class="Str"(reference=w142, error in=w143, "Value"=w141) -> (error out=w140:errorcluster)  [unwired: 1 out]
        }
        n93 = in-place-dvr #1(w104) -> (w76:refnum<data-value>)  [unwired: 1 out]
      }
      "# created images" <- w90
      "# disposed images" <- w87
      n94 = Merge Errors(w34, w36) -> (w33:errorcluster)
      n95 = Sort 1D Array(array=w54) -> (sorted array=w51:u8[])
      n96 = call "AlliGator Update Dataset Series Slide.vi"("Dataset Series Slide Ref"=w73, "Current Time Stamp Ref"=w74, "Error In"=w35, "Path"=w52, "Dataset Series Paths"=w71) -> ("Error Out"=w69:errorcluster)  [unwired: 5 in, 1 out]
      n97 = Reciprocal(x=w31) -> (1/x=w27:dbl[unit])
      n98 = call "AlliGator Harmonic Orders String.vi"("Harmonic Order Array"=w51) -> ("String"=w58:string)  [unwired: 8 in]
      n99 = Bundle By Name(cluster=T2 {"Nanotime Gate Separation"=nan, "Gate Width"=nan, "Laser Period"=nan, "Data Description"="", "# Pixel X"=-1, "# Pixel Y"=-1, "Gates to Use"={"Start"=0, "End"=0}, "Gate Step"=-1, "SYNC Period"=0.0, "X Binning"=0, "Y Binning"=0, "Gates to"=FALSE, "Metadata"="", "Gate Image Exposure"=0.0, "Gate Image Integration"=0.0, "Macrotime Gate Separation"=0.0}, "X Binning"=w26, "Y Binning"=w25, "# Pixel X"=w60, "# Pixel Y"=w59, "Laser Period"=w27, "Data Description"=w32, "SYNC Period"=w27) -> (w85:T2)
      n100 = call "Set Slide Range.vi"("Max"=w65, "error in (no error)"=w35, "Slide in"=w72) -> ("error out"=w68:errorcluster)  [unwired: 8 in]
      n101 = Merge Errors(w68, w69, w34) -> (w66:errorcluster)
      n102 = call "Clear Error.vi"("Error In"=w66) -> ()  [unwired: 8 in, 1 out]
      n103 = call "AlliGator Update Loaded Dataset Info.vi"("Image Loading Options"=w21, "Background File?"=w22, "Pile-up Correction"=FALSE, "error in (no error)"=w33, "After Loading Dataset Information"=w85, "# Gates"=w65, "Pixel Well Capacity"=u32 0) -> ("Error Out"=w84:errorcluster)  [unwired: 4 in]
      n104 = expression code="x/2"(w65) -> (w55:i32)
      n105 = Format Into String(format string="I/m/phi Dataset loaded: %s\n%s\n# Harmonics: %d  %s\n", error in=w84, w52, w82, w55, w58) -> (resulting string=w88:string, error out=w70:errorcluster)  [unwired: 1 in]
      "Folder Path (dup)" <- w52
    }
    frame True {
      n106 = xnode "Error Ring"() -> ("error out"=w478:errorcluster)
    }
  }
  "error out" <- w10
  "Result String" <- w11
  "AlliGator IV DVR out" <- w8
